vi "get tag index.vi"(8 "error in":errorcluster, 10 "tag name":string, 11 "tag collection in":refnum<class "tag collection.lvclass">) -> (0 "error out":errorcluster, 1 "index":i32, 3 "tag collection out":refnum<class "tag collection.lvclass">)   [LabVIEW 2013, in "tag bus.lvlib" / "tag collection.lvclass"]
uses:
  tag collection.lvclass
  tag collection.lvclass/tag collection.ctl
  dictionary/search/search string list.vi
  dictionary/search/binary search.lvlib
  tag bus.lvlib
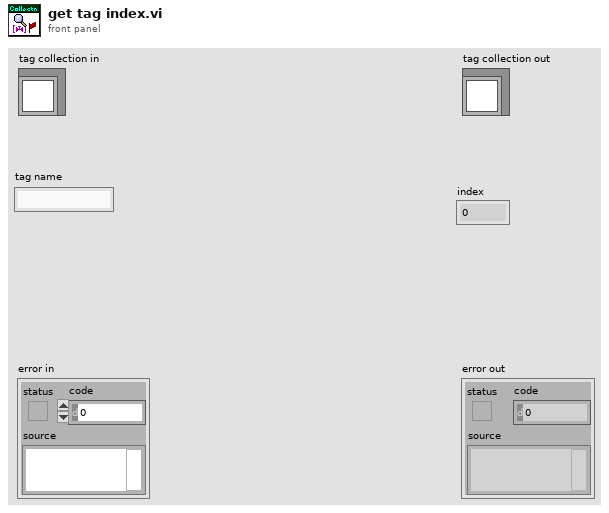
[diagram p1: front panel]
types:
  T1 = typedef "tag bus.lvlib/binary search.lvlib/sorted list.ctl" = cluster{"sorted strings":string[], "sorted indices":i32[]}
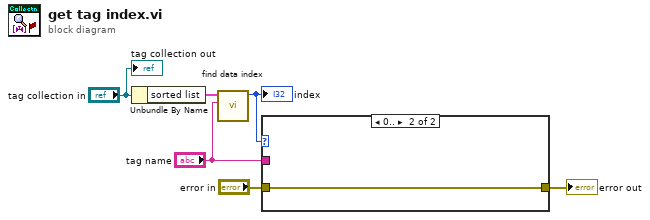
[diagram p0: block diagram]
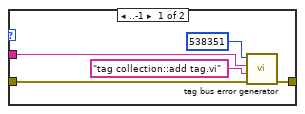
[diagram p2: hidden frame]
diagram:
  n1 = Unbundle By Name("tag collection in") -> ("sorted list"=w5:T1)
  n2 = call "find data index.vi"("string to locate"="tag name", "sorted list"=w5) -> ("index"=w4:i32)  [unwired: 9 in]
  "index" <- w4
  n3 = case shown="0.." w4 {
    tunnel: [w10 w12] -> w2
    tunnel: "error in" -> [w11 w12]
    tunnel: "tag name" -> [w7 _]
    frame ..-1 {
      n4 = call "tag bus error generator.vi"("error in"=w11, "source"="tag collection::add tag.vi", "append error message"=w7, "error code (0)"=538351) -> ("error out"=w10:errorcluster)  [unwired: 5 in]
    }
    frame 0.. {
    }
  }
  "error out" <- w2
  "tag collection out" <- "tag collection in"
